vi "display.vi"(8 "error in (no error)":errorcluster, 10 "OutcomeList.lvclass":refnum<class "OutcomeList.lvclass">, 11 "GoalUserInterface in":refnum<class "OutcomeListUIAdapter.lvclass">) -> (0 "error out":errorcluster, 3 "GoalUserInterface out":refnum<class "OutcomeListUIAdapter.lvclass">)   [LabVIEW 2018, in "OutcomeListUIAdapter.lvclass"]
uses:
  OutcomeListUIAdapter.lvclass
  OutcomeList/OutcomeList.lvclass
  OutcomeListUIAdapter.lvclass/OutcomeListUIAdapter.ctl
  <vilib>/Utility/miscctls.llb/LVRowAndColumnTypeDef.ctl
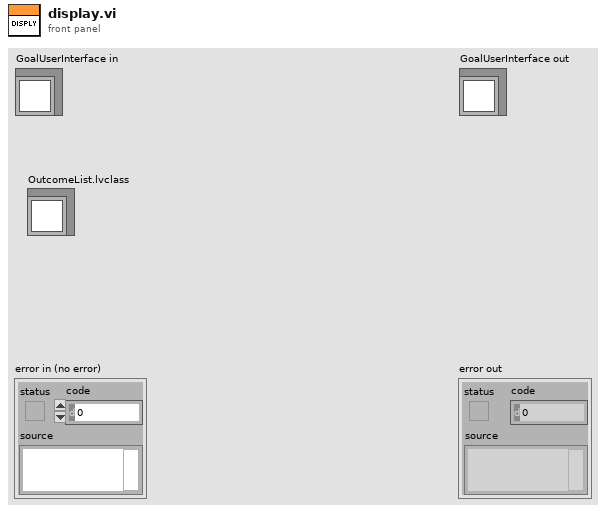
[diagram p1: front panel]
types:
  T1 = typedef "LVRowAndColumnTypeDef.ctl" = cluster{"Row":i32, "Column":i32}
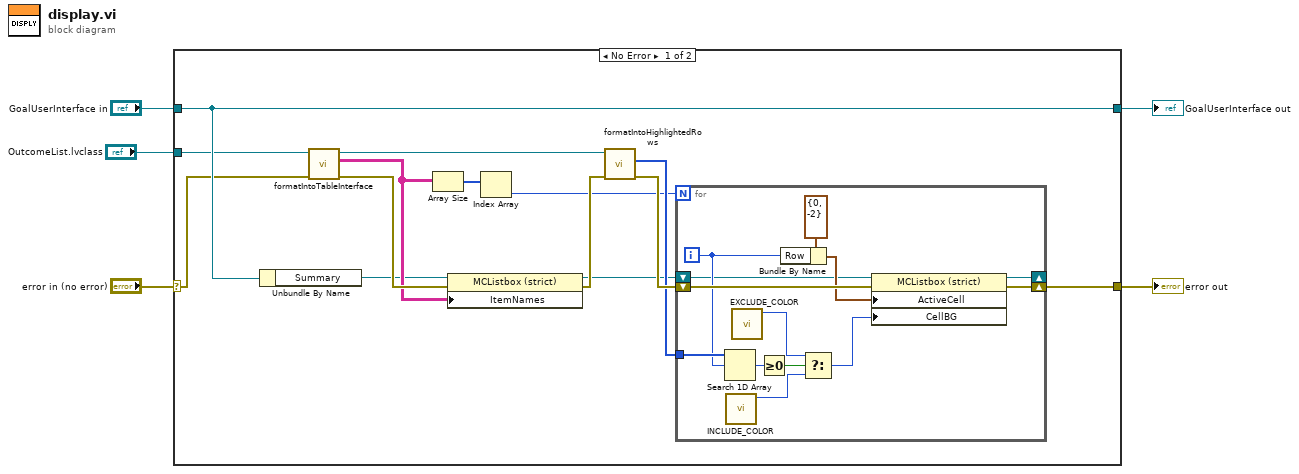
[diagram p0: block diagram]
diagram:
  n1 = case shown="No Error" "error in (no error)" {
    selector: "error in (no error)" -> [w7 w34]
    tunnel: [w6 w34] -> w4
    tunnel: [w9 w33] -> w2
    tunnel: "GoalUserInterface in" -> [w9 w33]
    tunnel: "OutcomeList.lvclass" -> [w8 _]
    frame No Error {
      n2 = Unbundle By Name(w9) -> ("Summary"=w12:refnum<vi>)
      n3 = call "formatIntoTableInterface.vi"("error in (no error)"=w7, "OutcomeList in"=w8) -> ("error out"=w15:errorcluster, "Table Interface"=w14:string[][], "OutcomeList out"=w16:refnum<class "OutcomeList.lvclass">)  [unwired: 7 in]
      n4 = Array Size(array=w14) -> (size(s)=w10:i32[])
      n5 = property on="Property Node" class="MCListbox (strict)"(reference=w12, error in=w15, "ItemNames"=w14) -> (reference out=w13:refnum<vi>, error out=w18:errorcluster)
      n6 = Index Array(array=w10) -> (element=w11:i32)  [unwired: 1 in]
      n7 = call "formatIntoHighlightedRows.vi"("error in (no error)"=w18, "OutcomeList in"=w16) -> ("error out"=w19:errorcluster, "Highlighted Rows"=w17:i32[])  [unwired: 7 in, 1 out]
      n8 = for {
        N: w11 -> [_]
        shift-right: [w31] -> w6
        shift-left: w19 -> [w32]
        tunnel: w17 -> [w27]
        shift-right: [w22] -> _
        shift-left: w13 -> [w23]
        i -> [w26]
        n9 = Search 1D Array(1D array=w27, element=w26) -> (index of element=w25:i32)  [unwired: 1 in]
        n10 = call "INCLUDE_COLOR.vi"() -> ("Color Box"=w20:u32)  [unwired: 11 in]
        n11 = call "EXCLUDE_COLOR.vi"() -> ("Color Box"=w21:u32)  [unwired: 11 in]
        n12 = Greater Or Equal To 0?(x=w25) -> (x >= 0?=w24:bool)
        n13 = Bundle By Name(cluster=T1 {"Row"=0, "Column"=-2} ("Active Cell:Active Cell"), "Row"=w26) -> (w28:T1)
        n14 = Select(t=w21, s=w24, f=w20) -> (s? t:f=w29:u32)
        n15 = property on="Property Node" class="MCListbox (strict)"(reference=w23, error in=w32, "ActiveCell"=w28, "CellBG"=w29) -> (reference out=w22:refnum<vi>, error out=w31:errorcluster)
      }
    }
    frame Error {
    }
  }
  "error out" <- w4
  "GoalUserInterface out" <- w2
